vi "Joystick Key To Displayed Arrow.vi"(5 "Joystick":T1) -> (2 "Color[]":u32[][](array[numeric]))   [LabVIEW 2020]
uses:
  globalArrows.vi
  src/RPI.SenseHat.Joystick/TypeDefs/Joystick.ctl
  src/RPI.SenseHat.Joystick/RPI.SenseHat.Joystick.lvlib
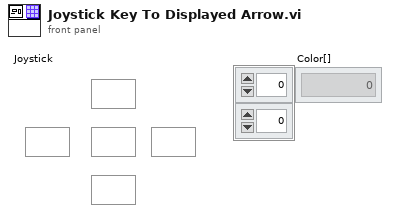
[diagram p1: front panel]
types:
  T1 = typedef "RPI.SenseHat.Joystick.lvlib/Joystick.ctl" = cluster{"Enter":bool, "Down":bool, "Up":bool, "Right":bool, "Left":bool}
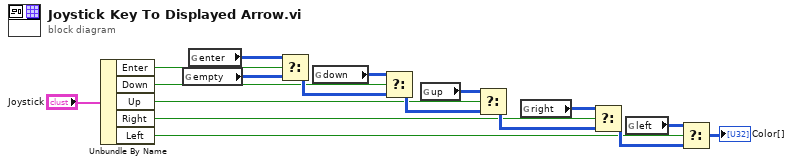
[diagram p0: block diagram]
diagram:
  n1 = Unbundle By Name("Joystick") -> ("Enter"=w2:bool, "Down"=w4:bool, "Up"=w6:bool, "Right"=w9:bool, "Left"=w10:bool)
  n2 = global read "globalArrows.vi" "empty"() -> (w16:u32[][])
  n3 = global read "globalArrows.vi" "enter"() -> (w3:u32[][])
  n4 = Select(t=w3, s=w2, f=w16) -> (s? t:f=w15:u32[][])
  n5 = global read "globalArrows.vi" "down"() -> (w5:u32[][])
  n6 = Select(t=w5, s=w4, f=w15) -> (s? t:f=w14:u32[][])
  n7 = global read "globalArrows.vi" "up"() -> (w7:u32[][])
  n8 = Select(t=w7, s=w6, f=w14) -> (s? t:f=w13:u32[][])
  n9 = global read "globalArrows.vi" "right"() -> (w8:u32[][])
  n10 = Select(t=w8, s=w9, f=w13) -> (s? t:f=w12:u32[][])
  n11 = global read "globalArrows.vi" "left"() -> (w11:u32[][])
  n12 = Select(t=w11, s=w10, f=w12) -> (s? t:f=→"Color[]":u32[][])
